vi "GenInstr-MainPopUp.vi"(7 "Raw Data From DB Actor":string[][](array[string]), 8 "error in (no error)":errorcluster, 11 "ERP-CreateInstructions in":refnum<class "ERP-CreateInstructions.lvclass">) -> (0 "error out":errorcluster, 3 "ERP-CreateInstructions out":refnum<class "ERP-CreateInstructions.lvclass">, 5 "Selected Instruction":string)   [LabVIEW 2013, in "ERP-CreateInstructions.lvclass"]
uses:
  ERP-CreateInstructions.lvclass
panel:
  in  "Cancel Button":bool
  in  "Select":bool
  in  "General Instructions":i32(listbox)
  # "Press to attached the selected\nInstruction to the current step"
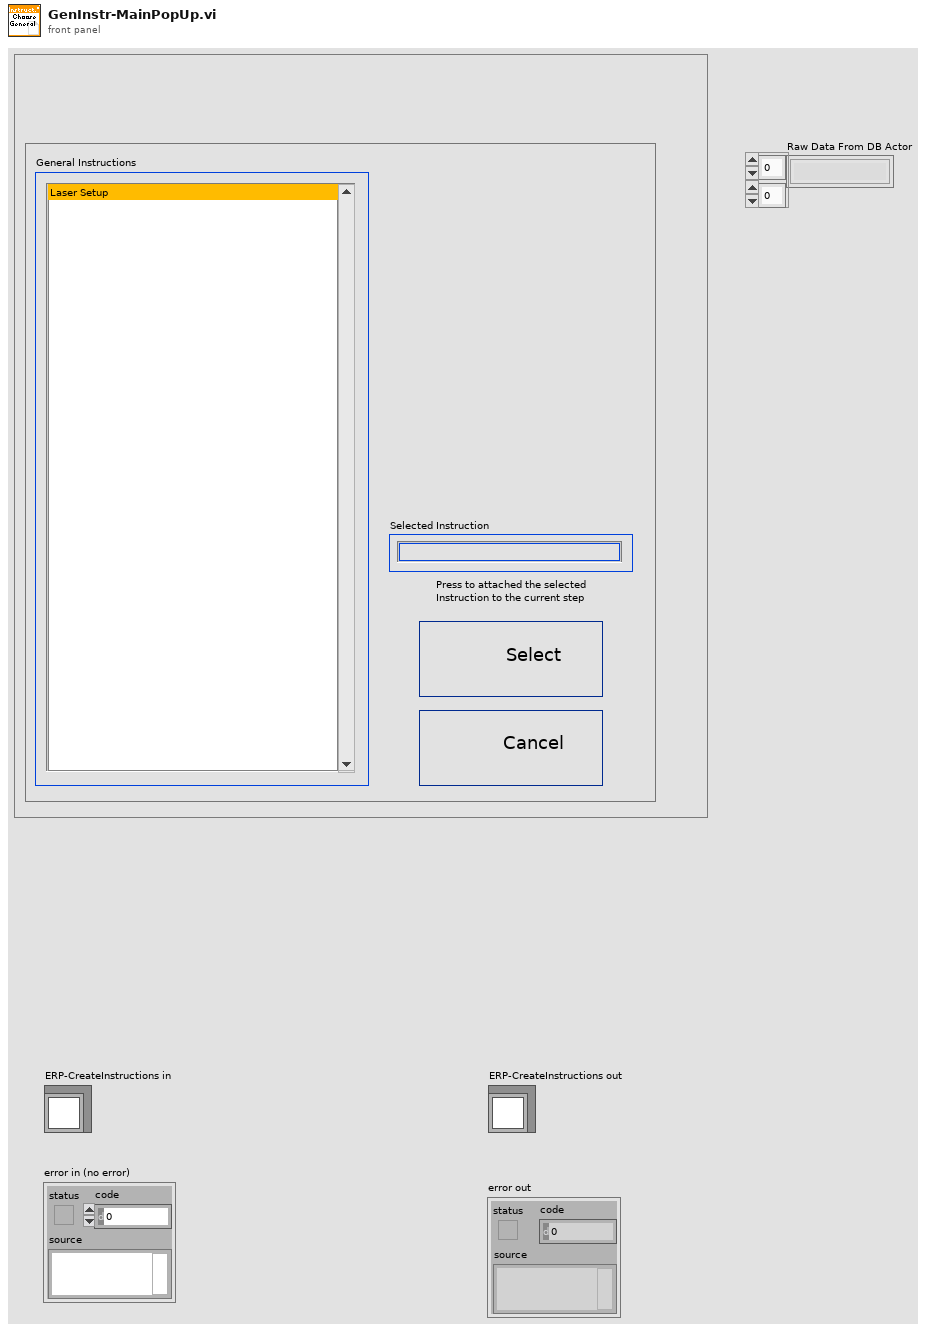
[diagram p1: front panel]
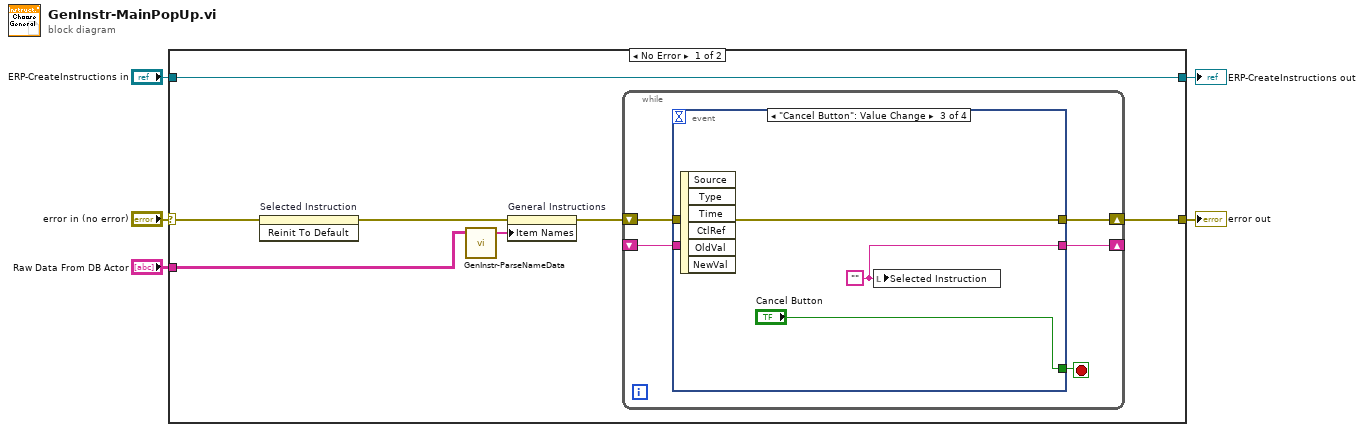
[diagram p0: block diagram]
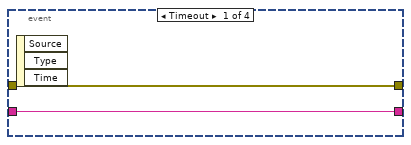
[diagram p2: hidden frame]
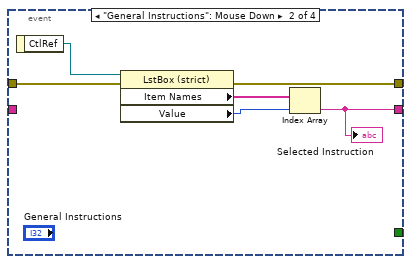
[diagram p3: hidden frame]
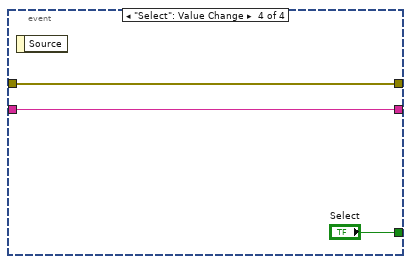
[diagram p4: hidden frame]
diagram:
  n1 = case shown="No Error" "error in (no error)" {
    selector: "error in (no error)" -> [w7 w33]
    tunnel: [w12 w33] -> w4
    tunnel: [w9 w32] -> w2
    tunnel: "ERP-CreateInstructions in" -> [w9 w32]
    tunnel: "Raw Data From DB Actor" -> [w8 _]
    frame No Error {
      n2 = invoke on="Selected Instruction" class="Str" method="Reinit To Default"(error in=w7) -> (error out=w6:errorcluster)  [unwired: 2 in, 2 out]
      n3 = call "GenInstr-ParseNameData.vi"("data"=w8) -> ("List of General Instructions"=w11:string[])  [unwired: 8 in]
      n4 = property on="General Instructions" class="LstBox (strict)"(error in=w6, "Item Names"=w11) -> (error out=w10:errorcluster)  [unwired: 1 in, 1 out]
      n5 = while {
        shift-right: [w16] -> w12
        shift-left: w10 -> [w17]
        shift-right: [w15] -> _
        shift-left: _ -> [w14]
        stop <- w13 stop-if-true
        n6 = event shown="[2] \"Cancel Button\": Value Change" {
          selector: _ -> [_ _ _ _]
          dyn-events: _ -> [_ _ _ _]
          timeout: _ -> [_ _ _ _]
          tunnel: w17 -> [w19 w25 w28 w31]
          tunnel: [w19 w21 w28 w31] -> w16
          tunnel: [w18 w20 w27 w30] -> w15
          tunnel: w14 -> [w18 _ _ w30]
          tunnel: [_ _ "Cancel Button" "Select"] -> w13
          event Timeout {
            n7 = event-data() -> ()  [unwired: 1 in, 3 out]
          }
          event "General Instructions": Mouse Down {
            n8 = event-data() -> ("CtlRef"=w24:refnum<vi>)  [unwired: 1 in]
            n9 = property class="LstBox (strict)"(reference=w24, error in=w25) -> (error out=w21:errorcluster, "Item Names"=w23:string[], "Value"=w22:i32)  [unwired: 1 out]
            n10 = Index Array(array=w23, index=w22) -> (element=w20:string)
            "Selected Instruction" <- w20
          }
          event "Cancel Button": Value Change {
            w27 = ""
            n11 = event-data() -> ()  [unwired: 1 in, 6 out]
            n12 = local write "Selected Instruction"(w27) -> ()
          }
          event "Select": Value Change {
            n13 = event-data() -> ()  [unwired: 1 in, 1 out]
          }
        }
      }
    }
    frame Error {
    }
  }
  "error out" <- w4
  "ERP-CreateInstructions out" <- w2
